vi "Realy Output Post Sub Steps Common LTT Signals.vi"(9 "Socket No":u16=1, 10 "RelayOutputWrite":T1, 11 "Sequence Context In":refnum<k7>) -> (0 "error out":errorcluster, 2 "PhysicalChannel":string[](array[string]), 3 "Report Text":string)   [LabVIEW 2023, in "LTT_TeststandSteptypes.lvlib"]
uses:
  LTT_TeststandSteptypes.lvlib
  Control/Relay Output.ctl
  <instrlib>/niSwitch/niSwitch.llb/niSwitch Topologies.ctl
  HardwareAbstractionLayer_LVOOP/NI Switch/NISwitch_class/NISwitch.lvclass
  <instrlib>/niSwitch/niSwitch.llb/niSwitch Relay Action.ctl
  HardwareAbstractionLayer_LVOOP/Digital Output/NI Digital Output_class/NI Digital Output.lvclass
  HardwareAbstractionLayer_LVOOP/Database/Database.lvclass
  HardwareAbstractionLayer_LVOOP/Database/SQL Public VI/Control/DB Options.ctl
panel:
  in  "error in":errorcluster
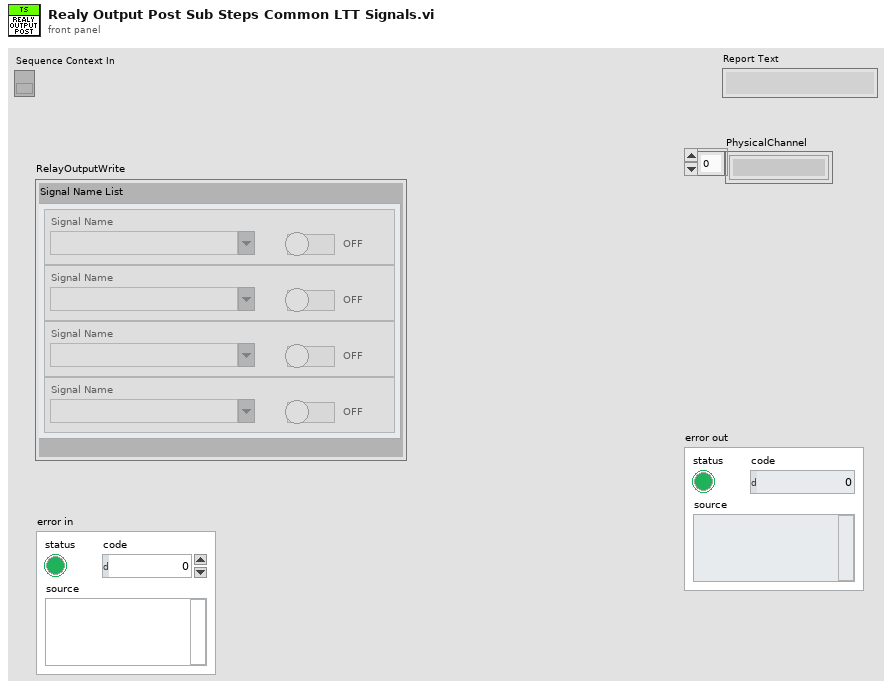
[diagram p1: front panel]
types:
  T1 = typedef "LTT_TeststandSteptypes.lvlib/Relay Output.ctl" = cluster{"Signal Name List":cluster{"Signal Name":string, "Enable Output":bool}[]}
  T2 = typedef "niSwitch Topologies.ctl" = string
  T3 = cluster{"Signal Name":string, "Enable Output":bool}[]
  T4 = typedef "HardwareAbstractionLayer_LVOOP.lvlib/Database.lvclass/DB Options.ctl" = enum16{"Init", "Select Data", "Insert Data", "Update Data", "Delete Data", "Execute Query", "Create Schema", "Create Table", "List Tables", "List Columns", "Close"}
  T5 = cluster{"table":string, "condition":string, "columns":string[]}
  T6 = typedef "niSwitch Relay Action.ctl" = i32
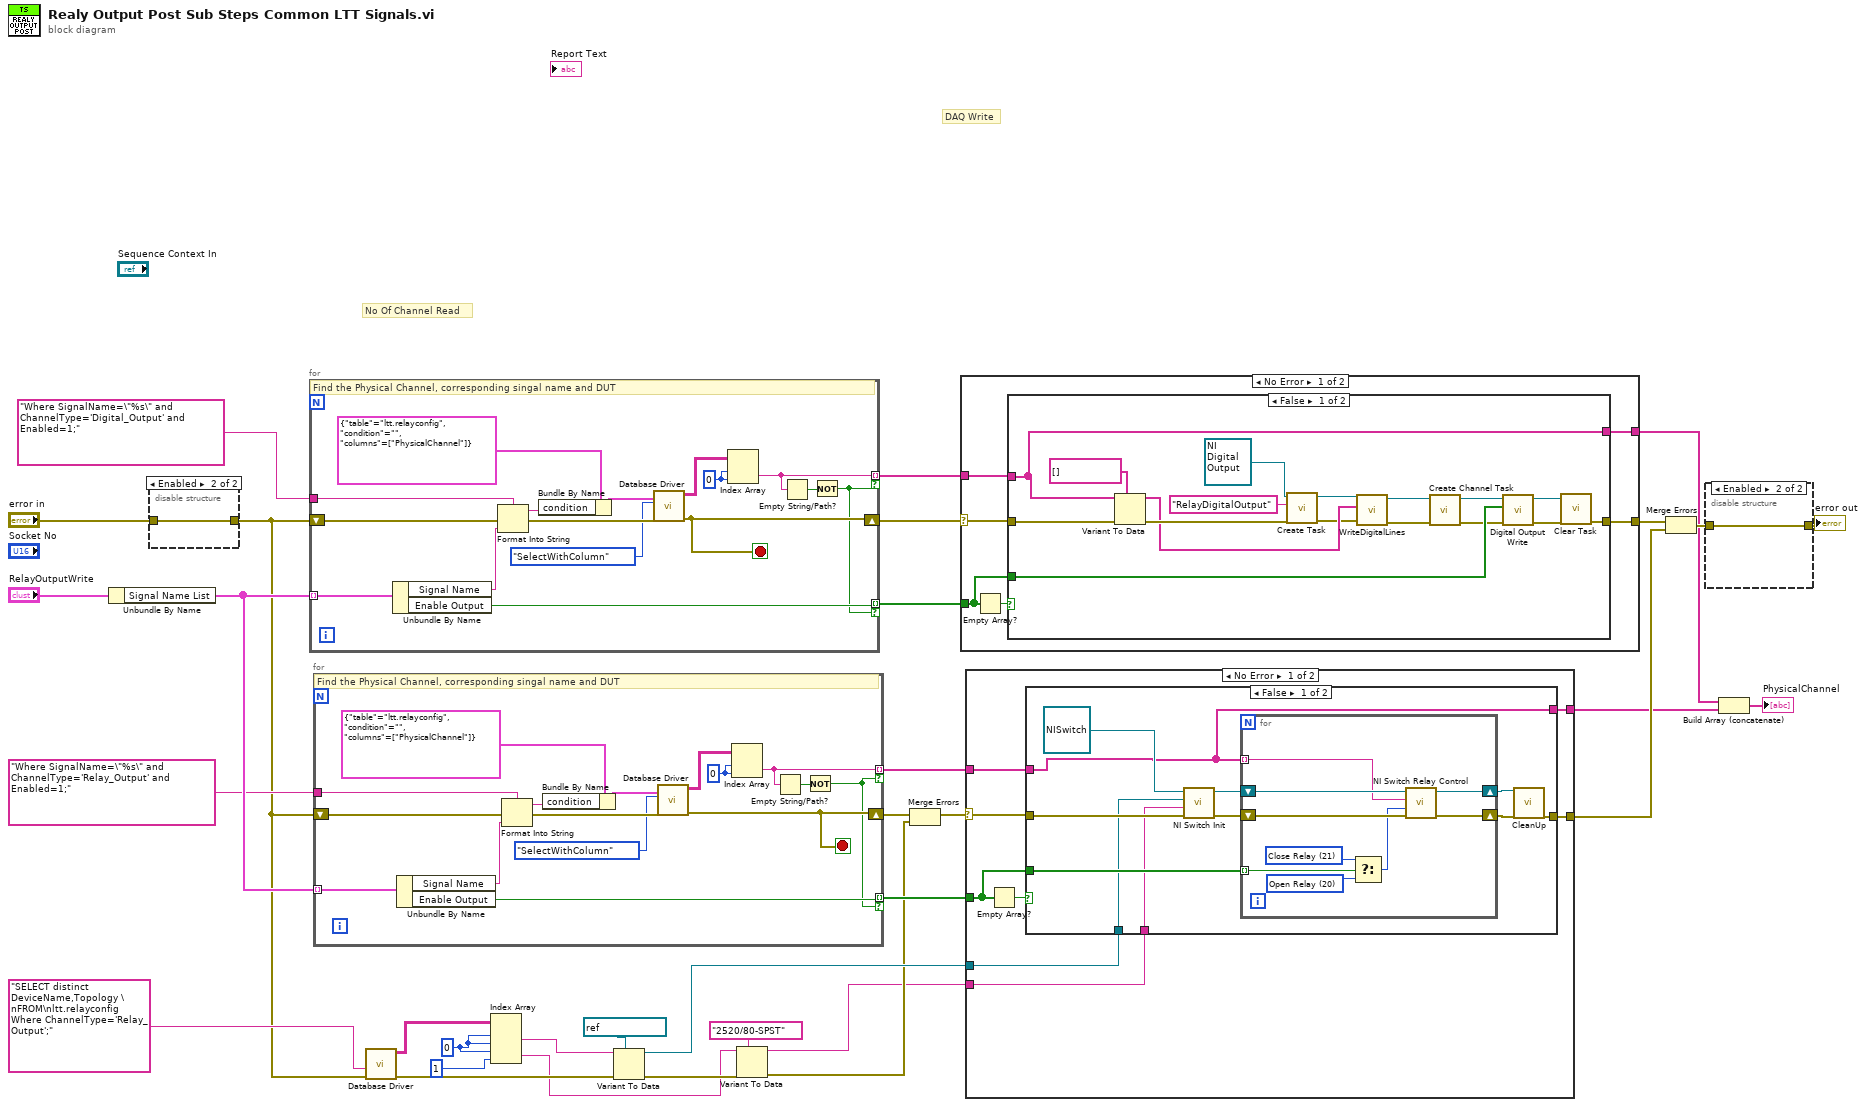
[diagram p0: block diagram]
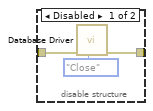
[diagram p2: hidden frame]
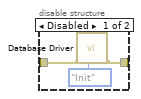
[diagram p3: hidden frame]
diagram:
  w13 = 0 ("disabled index (col)")
  # "DAQ Write"
  # "No Of Channel Read"
  n1 = Unbundle By Name("RelayOutputWrite") -> ("Signal Name List"=w27:T3)
  n2 = disable-structure shown="Enabled" {
    disable-tunnel: "error in" -> [w35 w37]
    disable-tunnel: [w34 w37] -> w6
    frame Disabled {
      n3 = call "Database Driver.vi"("Options"=DB_Options."Init", "error in"=w35) -> ("error out"=w34:errorcluster)  [unwired: 6 in, 3 out]
    }
    frame Enabled {
    }
  }
  n4 = for {
    tunnel: w27 -> [w44] mode=indexing
    tunnel: "Where SignalName=\"%s\" and ChannelType='Digital_Output' and Enabled=1;" -> [w53]
    shift-right: [w46] -> w30
    shift-left: w6 -> [w49]
    tunnel: [w42] -> w32 mode=indexing if=w38
    tunnel: [w40] -> w31 mode=indexing if=w38
    stop <- w46 stop-if-true
    w47 = 0 ("disabled index (col)")
    # "Find the Physical Channel, corresponding singal name and DUT"
    n5 = Unbundle By Name(w44) -> ("Signal Name"=w43:string, "Enable Output"=w42:bool)
    n6 = Format Into String(format string=w53, error in=w49, w43) -> (resulting string=w51:string, error out=w48:errorcluster)  [unwired: 1 in]
    n7 = Bundle By Name(cluster=T5 {"table"="ltt.relayconfig", "condition"="", "columns"=["PhysicalChannel"]} ("SQLTableData"), "condition"=w51) -> (w50:T5)
    n8 = call "Database Driver.vi"("SQLTableData"=w50, "error in"=w48, "Select"=enum16{"SelectWithQuery", "SelectWithColumn"}."SelectWithColumn") -> ("error out"=w46:errorcluster, "data"=w41:string[][])  [unwired: 5 in, 2 out]
    n9 = Index Array(array=w41, index (row)=w47, index (col)=w47) -> (element=w40:string)
    n10 = Empty String/Path?(string/path=w40) -> (empty?=w39:bool)
    n11 = Not(x=w39) -> (.not. x?=w38:bool)
  }
  n12 = for {
    tunnel: w27 -> [w61] mode=indexing
    shift-right: [w63] -> w26
    shift-left: w6 -> [w66]
    tunnel: [w59] -> w25 mode=indexing if=w54
    tunnel: [w55] -> w22 mode=indexing if=w54
    tunnel: "Where SignalName=\"%s\" and ChannelType='Relay_Output' and Enabled=1;" -> [w57]
    stop <- w63 stop-if-true
    w64 = 0 ("disabled index (col)")
    # "Find the Physical Channel, corresponding singal name and DUT"
    n13 = Unbundle By Name(w61) -> ("Signal Name"=w60:string, "Enable Output"=w59:bool)
    n14 = Format Into String(format string=w57, error in=w66, w60) -> (resulting string=w68:string, error out=w65:errorcluster)  [unwired: 1 in]
    n15 = Bundle By Name(cluster=T5 {"table"="ltt.relayconfig", "condition"="", "columns"=["PhysicalChannel"]} ("SQLTableData"), "condition"=w68) -> (w67:T5)
    n16 = call "Database Driver.vi"("SQLTableData"=w67, "error in"=w65, "Select"=enum16{"SelectWithQuery", "SelectWithColumn"}."SelectWithColumn") -> ("error out"=w63:errorcluster, "data"=w58:string[][])  [unwired: 5 in, 2 out]
    n17 = Index Array(array=w58, index (row)=w64, index (col)=w64) -> (element=w55:string)
    n18 = Empty String/Path?(string/path=w55) -> (empty?=w56:bool)
    n19 = Not(x=w56) -> (.not. x?=w54:bool)
  }
  n20 = call "Database Driver.vi"("error in"=w6, "SQL query"="SELECT distinct DeviceName,Topology \nFROM\nltt.relayconfig Where ChannelType='Relay_Output';") -> ("error out"=w19:errorcluster, "data"=w21:string[][])  [unwired: 6 in, 2 out]
  n21 = Index Array(array=w21, index (row) #1=w13, index (col) #1=w13, index (row) #2=w13, index (col) #2=1 ("disabled index (col)")) -> (element #1=w20:string, element #2=w17:string)
  n22 = Variant To Data(error in=w19, type=refnum<k15> "PXI2Slot17" ("resource name"), Variant=w20) -> (data=w11:refnum<k15>, error out=w18:errorcluster)
  n23 = Variant To Data(error in=w18, type=T2 "2520/80-SPST" ("topology name"), Variant=w17) -> (data=w8:T2, error out=w9:errorcluster)
  n24 = Merge Errors(w26, w9) -> (w10:errorcluster)
  n25 = case shown="No Error" w30 {
    selector: w30 -> [w73 w94]
    tunnel: w32 -> [w72 _]
    tunnel: w31 -> [w74 _]
    tunnel: [w71 w94] -> w28
    tunnel: [w70 _] -> w3
    frame No Error {
      n26 = Empty Array?(array=w72) -> (empty?=w75:bool)
      n27 = case shown="False" w75 {
        tunnel: w74 -> [w76 _]
        tunnel: w73 -> [w92 w93]
        tunnel: w72 -> [w84 _]
        tunnel: [w82 w93] -> w71
        tunnel: [w76 _] -> w70
        frame False {
          n28 = Variant To Data(error in=w92, type=tag[] [] ("DigitalLines"), Variant=w76) -> (data=w88:tag[], error out=w91:errorcluster)
          n29 = call-dynamic "Create Task.vi"("error in"=w91, "Task Name"="RelayDigitalOutput", "NI Digital Output in"=refnum<class "NI Digital Output.lvclass"> refnum ("HardwareAbstractionLayer_LVOOP.lvlib:NI Digital Output.lvclass")) -> ("error out"=w85:errorcluster, "NI Digital Output out"=w89:refnum<class "NI Digital Output.lvclass">)  [unwired: 7 in]
          n30 = call-dynamic "WriteDigitalLines.vi"("error in (no error)"=w85, "DigitalLines"=w88, "NI Digital Output in"=w89) -> ("error out"=w79:errorcluster, "NI Digital Output out"=w81:refnum<class "NI Digital Output.lvclass">)  [unwired: 7 in]
          n31 = call-dynamic "Create Channel Task.vi"("error in"=w79, "NI Digital Output in"=w81) -> ("error out"=w78:errorcluster, "NI Digital Output out"=w80:refnum<class "NI Digital Output.lvclass">)  [unwired: 8 in]
          n32 = call-dynamic "Digital Output Write.vi"("error in"=w78, "Digital Output Write"=w84, "NI Digital Output in"=w80) -> ("error out"=w77:errorcluster, "NI Digital Output out"=w83:refnum<class "NI Digital Output.lvclass">)  [unwired: 7 in]
          n33 = call-dynamic "Clear Task.vi"("error in"=w77, "NI Digital Output in"=w83) -> ("error out"=w82:errorcluster)  [unwired: 8 in, 1 out]
        }
        frame True {
        }
      }
    }
    frame Error {
    }
  }
  n34 = case shown="No Error" w10 {
    selector: w10 -> [w98 w124]
    tunnel: w25 -> [w101 _]
    tunnel: [w100 w124] -> w24
    tunnel: w22 -> [w99 _]
    tunnel: w11 -> [w97 _]
    tunnel: w8 -> [w96 _]
    tunnel: [w95 _] -> w2
    frame No Error {
      n35 = Empty Array?(array=w101) -> (empty?=w102:bool)
      n36 = case shown="False" w102 {
        tunnel: w98 -> [w112 w123]
        tunnel: w101 -> [w106 _]
        tunnel: [w107 w123] -> w100
        tunnel: w99 -> [w103 _]
        tunnel: w97 -> [w105 _]
        tunnel: w96 -> [w104 _]
        tunnel: [w103 _] -> w95
        frame False {
          n37 = call "NI Switch Init.vi"("error in (no error)"=w112, "topology name"=w104, "resource name"=w105, "object in"=refnum<class "NISwitch.lvclass"> refnum ("HardwareAbstractionLayer_LVOOP.lvlib:RelayOutput")) -> ("error out"=w110:errorcluster, "object out"=w111:refnum<class "NISwitch.lvclass">)  [unwired: 6 in]
          n38 = for {
            shift-right: [w120] -> w109
            shift-left: w111 -> [w122]
            shift-right: [w119] -> w108
            shift-left: w110 -> [w121]
            tunnel: w106 -> [w117] mode=indexing
            tunnel: w103 -> [w114] mode=indexing
            w116 = T6 20 items=["Open Relay"=20, "Close Relay"=21] ("f")
            w118 = T6 21 items=["Open Relay"=20, "Close Relay"=21] ("relay action (Close Relay)")
            n39 = Select(t=w118, s=w117, f=w116) -> (s? t:f=w115:T6)
            n40 = call-dynamic "NI Switch Relay Control.vi"("error in (no error)"=w121, "relay action (Close Relay)"=w115, "relay names"=w114, "RelayOutput in"=w122) -> ("error out"=w119:errorcluster, "RelayOutput out"=w120:refnum<class "NISwitch.lvclass">)  [unwired: 6 in]
          }
          n41 = call-dynamic "CleanUp.vi"("object in"=w109, "error in (no error)"=w108) -> ("error out"=w107:errorcluster)  [unwired: 16 in, 1 out]
        }
        frame True {
        }
      }
    }
    frame Error {
    }
  }
  n42 = Merge Errors(w28, w24) -> (w5:errorcluster)
  n43 = disable-structure shown="Enabled" {
    disable-tunnel: w5 -> [w127 w128]
    disable-tunnel: [w126 w128] -> w4
    frame Disabled {
      n44 = call "Database Driver.vi"("Options"=DB_Options."Close", "error in"=w127) -> ("error out"=w126:errorcluster)  [unwired: 6 in, 3 out]
    }
    frame Enabled {
    }
  }
  "error out" <- w4
  n45 = Build Array (concatenate)(w3, w2) -> (→"PhysicalChannel":string[])
